vi "read_write.vi"(10 "Enum":enum16{"read", "write"}(ring), 11 "command_in":string) -> (3 "command_out":string)   [LabVIEW 2018]
panel:
  out "write":string
  out "read":string
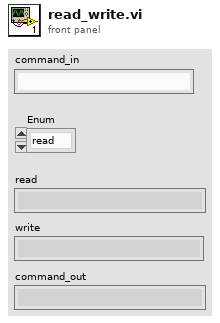
[diagram p1: front panel]
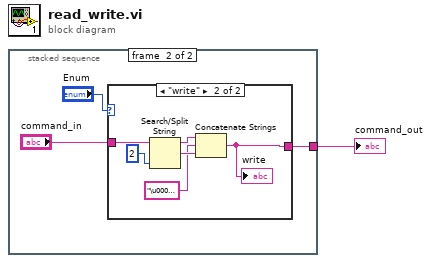
[diagram p0: block diagram]
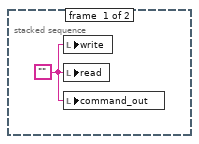
[diagram p2: hidden frame]
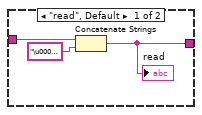
[diagram p3: hidden frame]
diagram:
  n1 = stacked-sequence {
    tunnel: [_ w3] -> w1
    frame #0 {
      w2 = ""
      n2 = local write "write"(w2) -> ()
      n3 = local write "read"(w2) -> ()
      n4 = local write "command_out"(w2) -> ()
    }
    frame #1 {
      n5 = case shown="\"write\"" "Enum" {
        tunnel: "command_in" -> [w8 w14]
        tunnel: [w6 w9] -> w3
        frame "read", Default {
          n6 = Concatenate Strings(w8, "\u0003\u0001" ("string")) -> (w6:string)
          "read" <- w6
        }
        frame "write" {
          n7 = Search/Split String(string=w14, offset (0)=2) -> (substring before match=w12:string, match + rest of string=w11:string)  [unwired: 1 in, 1 out]
          n8 = Concatenate Strings(w12, "\u0006\u0001" ("string"), w11) -> (w9:string)
          "write" <- w9
        }
      }
    }
  }
  "command_out" <- w1
